vi "Read Nodes.vi"(8 "error in (no error)":errorcluster, 11 "abs_Composite in":refnum<class "abs_Composite.lvclass">) -> (0 "error out":errorcluster, 2 "Nodes":refnum<class "abs_Node.lvclass">[](array[class]), 3 "abs_Composite out":refnum<class "abs_Composite.lvclass">)   [LabVIEW 2021, in "BT.lvlib" / "abs_Composite.lvclass"]
uses:
  abs_Composite.lvclass
  abs_Node/abs_Node.lvclass
  abs_Composite.lvclass/abs_Composite.ctl
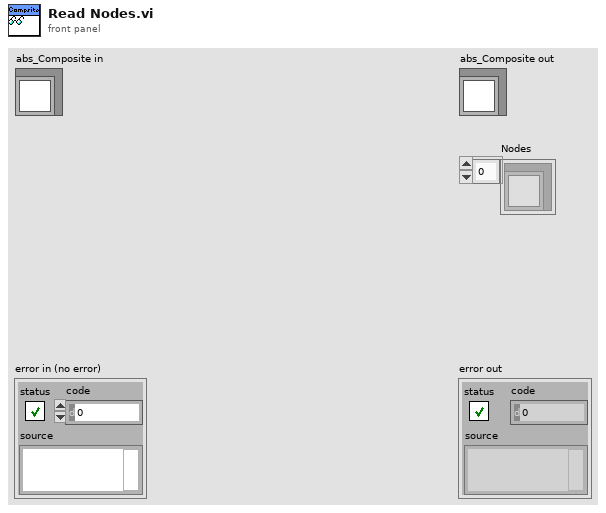
[diagram p1: front panel]
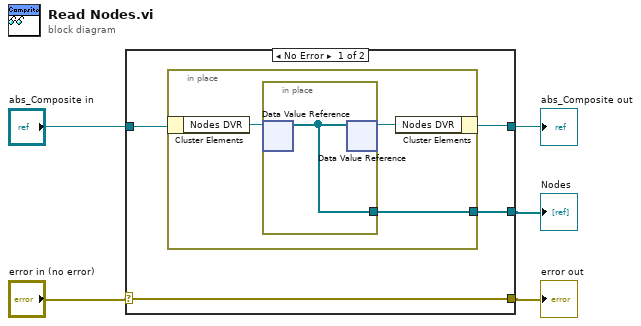
[diagram p0: block diagram]
diagram:
  n1 = case shown="No Error" "error in (no error)" {
    selector: "error in (no error)" -> [w9 w14]
    tunnel: [w9 w14] -> w1
    tunnel: [w6 w15] -> w3
    tunnel: "abs_Composite in" -> [w8 w15]
    tunnel: [w7 _] -> w2
    frame No Error {
      n2 = in-place {
        in-place-border: [w10] -> w7
        n3 = in-place-cluster #1(w8) -> ("Nodes DVR"=w12:refnum<data-value>)
        n4 = in-place {
          in-place-border: [w13] -> w10
          n5 = in-place-dvr #2(w12) -> (w13:refnum<class "abs_Node.lvclass">[])  [unwired: 1 out]
          n6 = in-place-dvr #2(w13) -> (w11:refnum<data-value>)  [unwired: 1 out]
        }
        n7 = in-place-cluster #1("Nodes DVR"=w11) -> (w6:refnum<class "abs_Composite.lvclass">)
      }
    }
    frame Error {
    }
  }
  "error out" <- w1
  "abs_Composite out" <- w3
  "Nodes" <- w2
